vi "ep_Energy Accumulation.vi"(0 "energy values":T1, 1 "restart (F)":bool, 7 "interval length (s)":dbl, 11 "error in (no error)":errorcluster) -> (4 "accumulated energy":T1, 8 "accumulation length (s)":dbl, 15 "error out":errorcluster)   [LabVIEW 2011, in "NI_EP_Power Quality.lvlib"]
doc: "This VI accumulates the energy values."
uses:
  <vilib>/addons/Electrical Power/PQ/NI_EP_Power Quality.lvlib
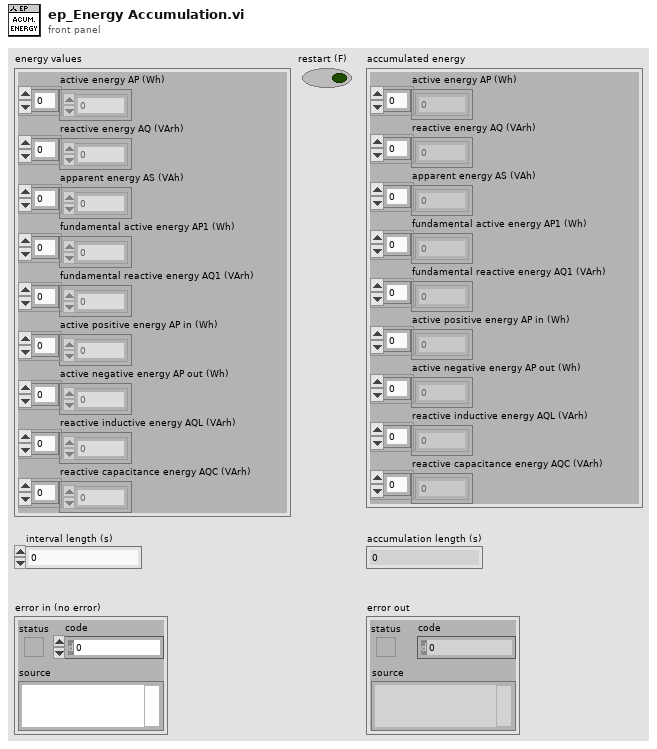
[diagram p1: front panel]
types:
  T1 = cluster{"active energy AP (Wh)":dbl[], "reactive energy AQ (VArh)":dbl[], "apparent energy AS (VAh)":dbl[], "fundamental active energy AP1 (Wh)":dbl[], "fundamental reactive energy AQ1 (VArh)":dbl[], "active positive energy AP in (Wh)":dbl[], "active negative energy AP out (Wh)":dbl[], "reactive inductive energy AQL (VArh)":dbl[], "reactive capacitance energy AQC (VArh)":dbl[]}
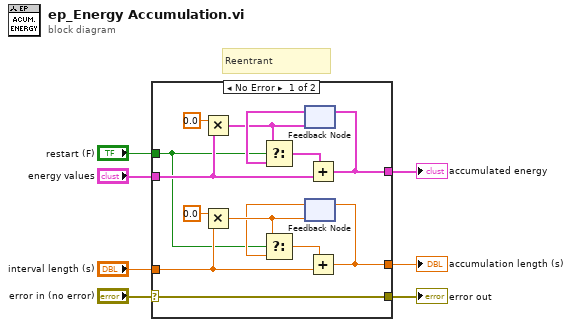
[diagram p0: block diagram]
diagram:
  # "Reentrant"
  n1 = case shown="No Error" "error in (no error)" {
    selector: "error in (no error)" -> [w8 w22]
    tunnel: "energy values" -> [w21 _]
    tunnel: [w19 _] -> w6
    tunnel: "interval length (s)" -> [w11 _]
    tunnel: "restart (F)" -> [w10 _]
    tunnel: [w9 _] -> w3
    tunnel: [w8 w22] -> w1
    frame No Error {
      n2 = Multiply(x=0.0, y=w21) -> (x*y=w17:T1)
      n3 = Multiply(x=0.0, y=w11) -> (x*y=w14:dbl)
      n4 = feedback #1(w17) -> (w18:T1)
      n5 = Select(t=w17, s=w10, f=w18) -> (s? t:f=w16:T1)
      n6 = feedback #2(w14) -> (w13:dbl)
      n7 = Select(t=w14, s=w10, f=w13) -> (s? t:f=w15:dbl)
      n8 = Add(x=w16, y=w21) -> (x+y=w19:T1)
      n9 = feedback-in #1(w19) -> ()
      n10 = Add(x=w15, y=w11) -> (x+y=w9:dbl)
      n11 = feedback-in #2(w9) -> ()
    }
    frame Error {
    }
  }
  "accumulated energy" <- w6
  "error out" <- w1
  "accumulation length (s)" <- w3
